vi "Write Multiple Input Registers.vi"(8 "error in (no error)":errorcluster, 9 "input register values":u16[](array[numeric]), 10 "starting address":u16, 11 "MB CR in":refnum<class "Modbus Master CR API.lvclass">) -> (0 "error out":errorcluster, 3 "MB CR out":refnum<class "Modbus Master CR API.lvclass">)   [LabVIEW 2021, in "Modbus Master CR API.lvclass"]
doc: "Writes values to multiple contiguous input registers."
uses:
  Modbus Master CR API.lvclass
  D:/my_projects/projects/Algorithms/Labview/21/Modbus_v121c/API/Modbus API.lvclass
  Modbus API.lvclass/Modbus API.ctl
  Network Protocol/MB/Modbus Master CR.lvclass/Modbus Master CR.ctl
  Read Network Protocol.vi
  Network Protocol/MB/Modbus Master CR.lvclass
  Data Model/Device Data Model.lvclass
  Modbus Master CR API.lvclass/Modbus Master CR API.ctl
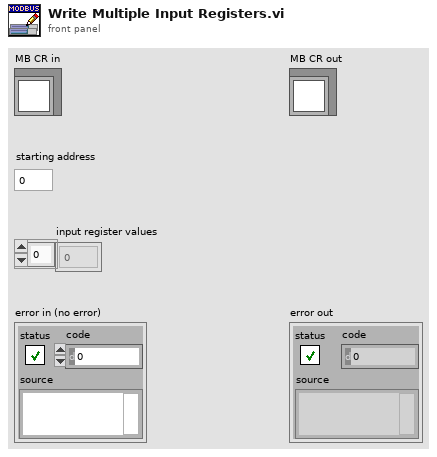
[diagram p1: front panel]
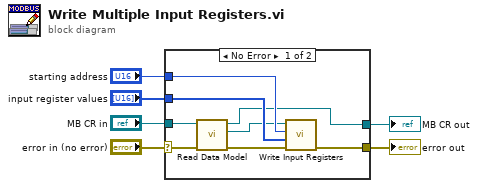
[diagram p0: block diagram]
diagram:
  n1 = case shown="No Error" "error in (no error)" {
    selector: "error in (no error)" -> [w11 w16]
    tunnel: [w12 w16] -> w4
    tunnel: "MB CR in" -> [w8 w15]
    tunnel: "input register values" -> [w14 _]
    tunnel: "starting address" -> [w13 _]
    tunnel: [w7 w15] -> w1
    frame No Error {
      n2 = call "Read Data Model.vi"("error in (no error)"=w11, "MB CR in"=w8) -> ("error out"=w10:errorcluster, "device data model"=w9:refnum<class "Device Data Model.lvclass">, "MB CR out"=w7:refnum<class "Modbus Master CR API.lvclass">)  [unwired: 7 in]
      n3 = call-dynamic "Write Input Registers.vi"("error in (no error)"=w10, "register values"=w14, "starting address"=w13, "Device Data Model in"=w9) -> ("error out"=w12:errorcluster)  [unwired: 6 in, 1 out]
    }
    frame Error {
    }
  }
  "error out" <- w4
  "MB CR out" <- w1
